vi "Close Client.vi"(8 "error in (no error)":errorcluster, 11 "Messaging Server Client in":refnum<class "Messaging Server Client.lvclass">) -> (0 "error out":errorcluster, 3 "Messaging Server Client out":refnum<class "Messaging Server Client.lvclass">)   [LabVIEW 2020, in "Volatus.lvlib" / "Messaging Server Client.lvclass"]
uses:
  Messaging Server Client.lvclass
  Messaging Server Client.lvclass/Messaging Server Client.ctl
  Module/Module.lvclass
  Volatus.lvlib
  C:/dev/lv20CE/relink/lv-volatus/Volatus/Module/Module.lvclass
  C:/dev/lv20CE/relink/lv-volatus/Volatus/Messaging Client/Messaging Server Client.lvclass
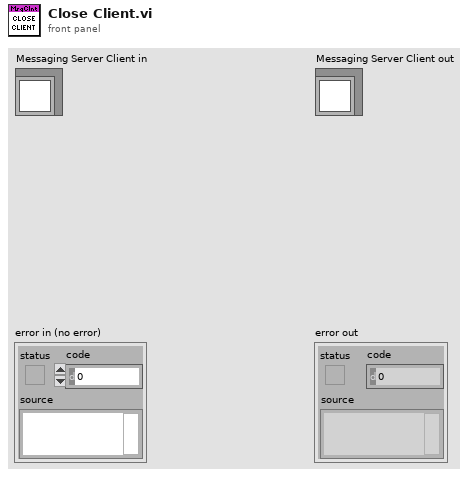
[diagram p1: front panel]
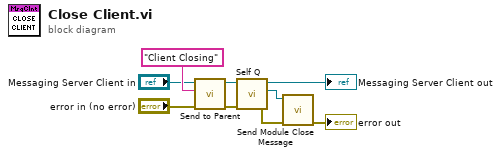
[diagram p0: block diagram]
diagram:
  n1 = call "Send to Parent.vi"("error in (no error)"="error in (no error)", "Message ID"="Client Closing", "Module in"="Messaging Server Client in") -> ("error out"=w5:errorcluster, "Module out"=w3:refnum<class "Messaging Server Client.lvclass">)  [unwired: 7 in]
  n2 = call "Self Q.vi"("Module in"=w3) -> ("Self Q"=w2:refnum<class "MessageQ.lvclass">, "Module out"=→"Messaging Server Client out":refnum<class "Messaging Server Client.lvclass">)  [unwired: 9 in]
  n3 = call "Send Module Close Message.vi"("error in (no error)"=w5, "MessageQ"=w2) -> ("error out"=→"error out":errorcluster)  [unwired: 9 in]
